vi "use rsa key data.vi"(8 "error in":errorcluster, 9 "format":i32, 10 "rsa key":string, 11 "connection creator in":refnum<class "connection creator.lvclass">) -> (0 "error out":errorcluster)   [LabVIEW 2016, in "connection creator.lvclass"]
uses:
  connection creator.lvclass
  connection creator.lvclass/connection creator.ctl
  dllwrapper/async tls dl.lvlib
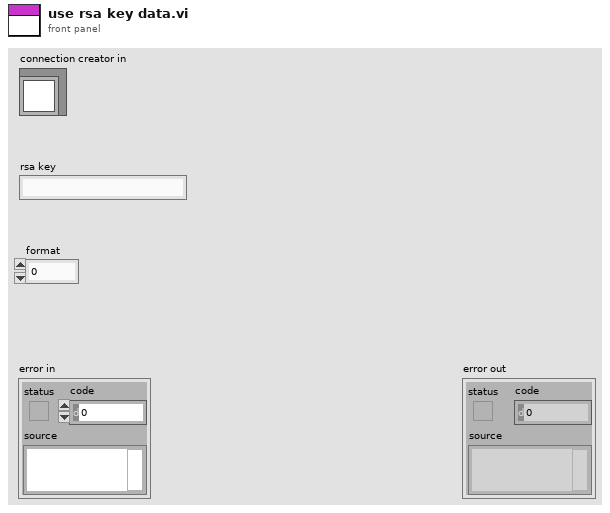
[diagram p1: front panel]
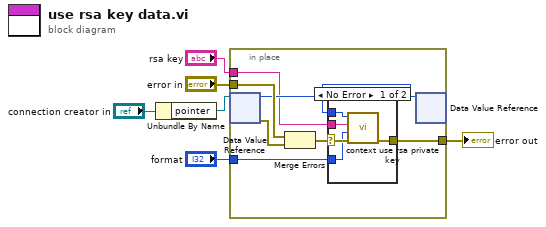
[diagram p0: block diagram]
diagram:
  n1 = Unbundle By Name("connection creator in") -> ("pointer"=w4:refnum<data-value>)
  n2 = in-place {
    in-place-border: "error in" -> [w12]
    in-place-border: [w10] -> w3
    in-place-border: "rsa key" -> [w8]
    in-place-border: "format" -> [w7]
    n3 = in-place-dvr #1(w4) -> (w9:u64, w13:errorcluster)
    n4 = Merge Errors(w12, w13) -> (w11:errorcluster)
    n5 = case shown="No Error" w11 {
      selector: w11 -> [w18 w19]
      tunnel: [w16 w19] -> w10
      tunnel: w9 -> [w17 _]
      tunnel: w8 -> [w15 _]
      tunnel: w7 -> [w14 _]
      frame No Error {
        n6 = call "context use rsa private key.vi"("error in"=w18, "format"=w14, "certificate data"=w15, "connector"=w17) -> ("error out"=w16:errorcluster)  [unwired: 7 in]
      }
      frame Error {
      }
    }
    n7 = in-place-dvr #1(w9) -> ()  [unwired: 2 out]
  }
  "error out" <- w3
